vi "Check-Characteristics-storage.vi"(8 "error in":errorcluster, 10 "Analysis params. ref.":refnum<data-value>, 11 "Save?":bool) -> (0 "error IO":errorcluster, 3 "Passed?":bool)   [LabVIEW 2013, in "CameraVision.lvlib" / "CV-Storage.lvclass"]
uses:
  CV-Storage.lvclass
  Analysis/CV-Analysis.lvclass
  Analysis/CV-Analysis.lvclass/CV-Analysis.ctl
  Analysis/Read Melt-pool characteristics.vi
  Analysis/Read Image characteristics.vi
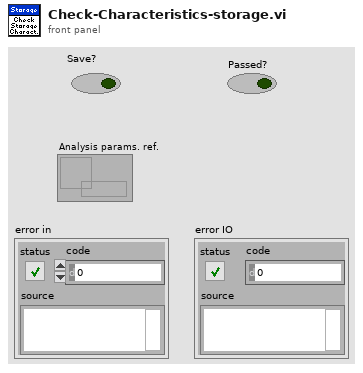
[diagram p1: front panel]
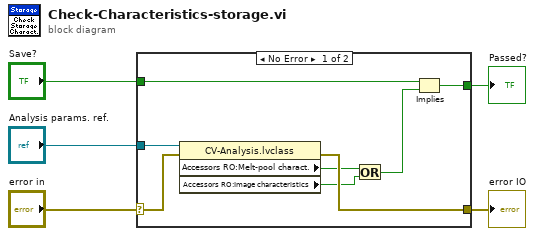
[diagram p0: block diagram]
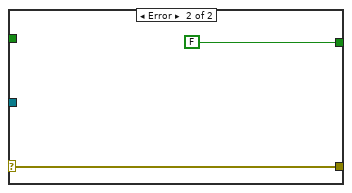
[diagram p2: hidden frame]
diagram:
  n1 = case shown="No Error" "error in" {
    selector: "error in" -> [w10 w14]
    tunnel: [w9 w14] -> w4
    tunnel: [w13 FALSE] -> w5
    tunnel: "Save?" -> [w12 _]
    tunnel: "Analysis params. ref." -> [w11 _]
    frame No Error {
      n2 = property class="CV-Analysis.lvclass"(reference=w11, error in=w10) -> (error out=w9:errorcluster, "Accessors RO:Melt-pool charact."=w8:bool, "Accessors RO:Image characteristics"=w7:bool)  [unwired: 1 out]
      n3 = Or(x=w8, y=w7) -> (x .or. y?=w6:bool)
      n4 = Implies(1:w6, 2:w12) -> (0:w13:bool)
    }
    frame Error {
    }
  }
  "Passed?" <- w5
  "error IO" <- w4
